vi "REQ Over Voltage Limit.vi"(8 "error in":errorcluster, 10 "Over Voltage Setting":T1) -> (0 "error out":errorcluster)   [LabVIEW 2016, in "DC PWS.lvlib"]
doc: "_____\nCreated using DQMH Event Scripter 6.1.0.128."
uses:
  DC PWS.lvlib
  REQ Over Voltage Limit Argument--cluster.ctl
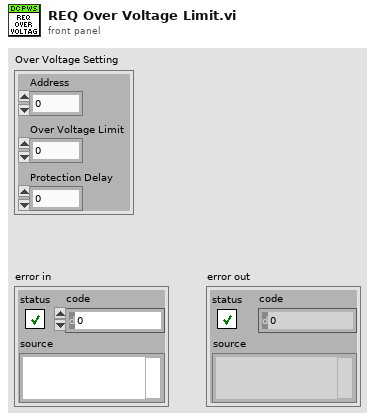
[diagram p1: front panel]
types:
  T1 = cluster{"Address":dbl, "Over Voltage Limit":dbl, "Protection Delay":dbl}
  T2 = typedef "DC PWS.lvlib/REQ Over Voltage Limit Argument--cluster.ctl" = cluster{"Over Voltage Setting":cluster{"Address":dbl, "Over Voltage Limit":dbl, "Protection Delay":dbl}}
  T3 = typedef "DC PWS.lvlib/Request Events--cluster.ctl" = cluster{"Stop Module":refnum<user-event>, "Show Panel":refnum<user-event>, "Hide Panel":refnum<user-event>, "Get Module Execution Status":refnum<user-event>, "Show Diagram":refnum<user-event>, "REQ Initialize Hardware":refnum<user-event>, "REQ Config Current Limit":refnum<user-event>, "REQ Over Voltage Limit":refnum<user-event>, "REQ Configure Output":refnum<user-event>, "REQ Enable Output":refnum<user-event>, "REQ Measurement":refnum<user-event>, "REQ Close Ref":refnum<user-event>, "REQ Wakeup_help_loop":refnum<user-event>, "REQ DC Parameter":refnum<user-event>, "REQ Retry DC PWS":refnum<user-event>}
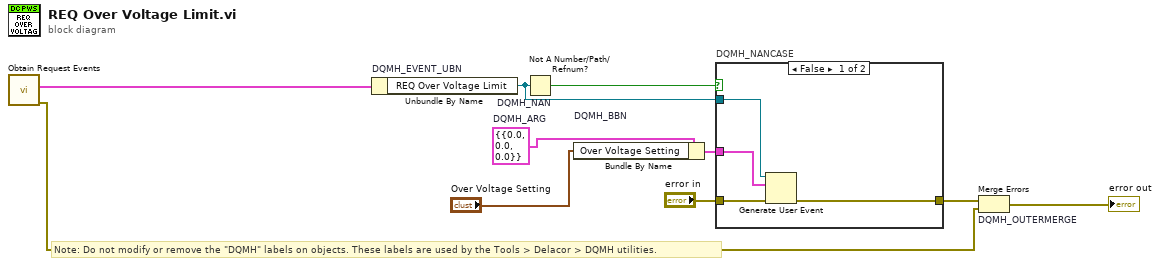
[diagram p0: block diagram]
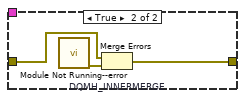
[diagram p2: hidden frame]
diagram:
  w4 = T2 {"Over Voltage Setting"={"Address"=0.0, "Over Voltage Limit"=0.0, "Protection Delay"=0.0}}  # DQMH_ARG
  # "Note: Do not modify or remove the \"DQMH\" labels on objects. These labels are used by the Tools > Delacor > DQMH utilities."
  n1 = call "Obtain Request Events.vi"() -> ("error out"=w2:errorcluster, "DC PWS Request Events"=w1:T3)  [unwired: 10 in]
  n2 = Unbundle By Name "DQMH_EVENT_UBN"(w1) -> ("REQ Over Voltage Limit"=w6:refnum<user-event>)
  n3 = Not A Number/Path/Refnum? "DQMH_NAN"(number/path/refnum=w6) -> (NaN/Path/Refnum?=w7:bool)
  n4 = Bundle By Name "DQMH_BBN"(cluster=w4, "Over Voltage Setting"="Over Voltage Setting") -> (w8:T2)
  n5 = case "DQMH_NANCASE" shown="False" w7 {
    tunnel: "error in" -> [w14 w17]
    tunnel: [w13 w16] -> w5
    tunnel: w6 -> [w12 _]
    tunnel: w8 -> [w11 _]
    frame False {
      n6 = Generate User Event(user event=w12, event data cluster=w11, error in=w14) -> (error out=w13:errorcluster)  [unwired: 1 in, 1 out]
    }
    frame True {
      n7 = call "Module Not Running--error.vi"() -> ("error out"=w15:errorcluster)  [unwired: 11 in]
      n8 = Merge Errors "DQMH_INNERMERGE"(w17, w15) -> (w16:errorcluster)
    }
  }
  n9 = Merge Errors "DQMH_OUTERMERGE"(w5, w2) -> (→"error out":errorcluster)
